vi "总磷总氮断电保存全局变量.vi"() -> ()   [LabVIEW 2022 SP3, in "斯坦道氨氮V2.lvlib"]
panel:
  in  "命令格式":u16(ring)=2 items=["自动", "低位在前", "低位在后"]
  in  "波特率":u32(ring)=115200 items=["115200"=115200, "9600"=9600]
  in  "低量程上限":cluster{"总磷":dbl, "总氮":dbl, "氨氮":dbl}={"总磷"=1.0, "总氮"=10.0, "氨氮"=1.0}
  out "总氮消解温度":dbl=120.0 caption="消解时长："
  out "总磷消解温度":dbl=120.0 caption="消解时长："
  out "校准条件":cluster{"线性相关系数":dbl}={"线性相关系数"=0.999}
  out "总氮消解时长":dbl=30.0 caption="消解时长："
  out "总磷消解时长":dbl=30.0 caption="消解时长："
  in  "盐度自动补偿：":bool
  out "启动队列名称":cluster{"String":string, "Value":u16}[](array[cluster])
  in  "氨氮自动测试量程配置":T1={"水样测试量程模式"=enum."AUTO", "空白核查量程模式"=enum."AUTO", "跨度核查量程模式"=enum."AUTO", "加标回收量程模式"=enum."AUTO", "标样核查量程模式"=enum."AUTO"}
  in  "MB通信方式选择":enum16{"串口", "TCP"}(ring)
  in  "PORT":string="502"
  in  "IP":string
  in  "VISA Resource":refnum<visa-resource-name>
  in  "运行周期":T2={"运行模式"=enum."维护模式", "质控频次"=enum."关闭", "空白核查时间"=2, "跨度核查时间"=6, "测量间隔"=240.0} {"跨度核查时间" items=["00H", "01H", "02H", "03H", "04H", "05H", "06H", "07H", "08H", "09H", "10H", "11H", "12H", "13H", "14H", "15H", "16H", "17H", "18H", "19H", "20H", "21H", "22H", "23H", "关闭"]; "空白核查时间" items=["00H", "01H", "02H", "03H", "04H", "05H", "06H", "07H", "08H", "09H", "10H", "11H", "12H", "13H", "14H", "15H", "16H", "17H", "18H", "19H", "20H", "21H", "22H", "23H", "关闭"]}
  in  "流程路径":path=path "data/流程.xml"
  in  "总氮自动测试量程配置":T1={"水样测试量程模式"=enum."AUTO", "空白核查量程模式"=enum."AUTO", "跨度核查量程模式"=enum."AUTO", "加标回收量程模式"=enum."AUTO", "标样核查量程模式"=enum."AUTO"}
  in  "质控参数设置":T3
  in  "总磷自动测试量程配置":T1={"水样测试量程模式"=enum."AUTO", "空白核查量程模式"=enum."AUTO", "跨度核查量程模式"=enum."AUTO", "加标回收量程模式"=enum."AUTO", "标样核查量程模式"=enum."AUTO"}
  # "℃"
  # "℃"
  # "min"
  # "min"
  # "运行模式："
  # "质控频次："
  # "零点核查时间："
  # "跨度核查时间："
  # "质控参数设置"
  # "总氮"
  # "氨氮"
  # "监测参数"
  # "总磷"
  # "跨度值"
  # "零点核查标准液浓度"
  # "跨度核查标准液浓度"
  # "标样核查标准液浓度"
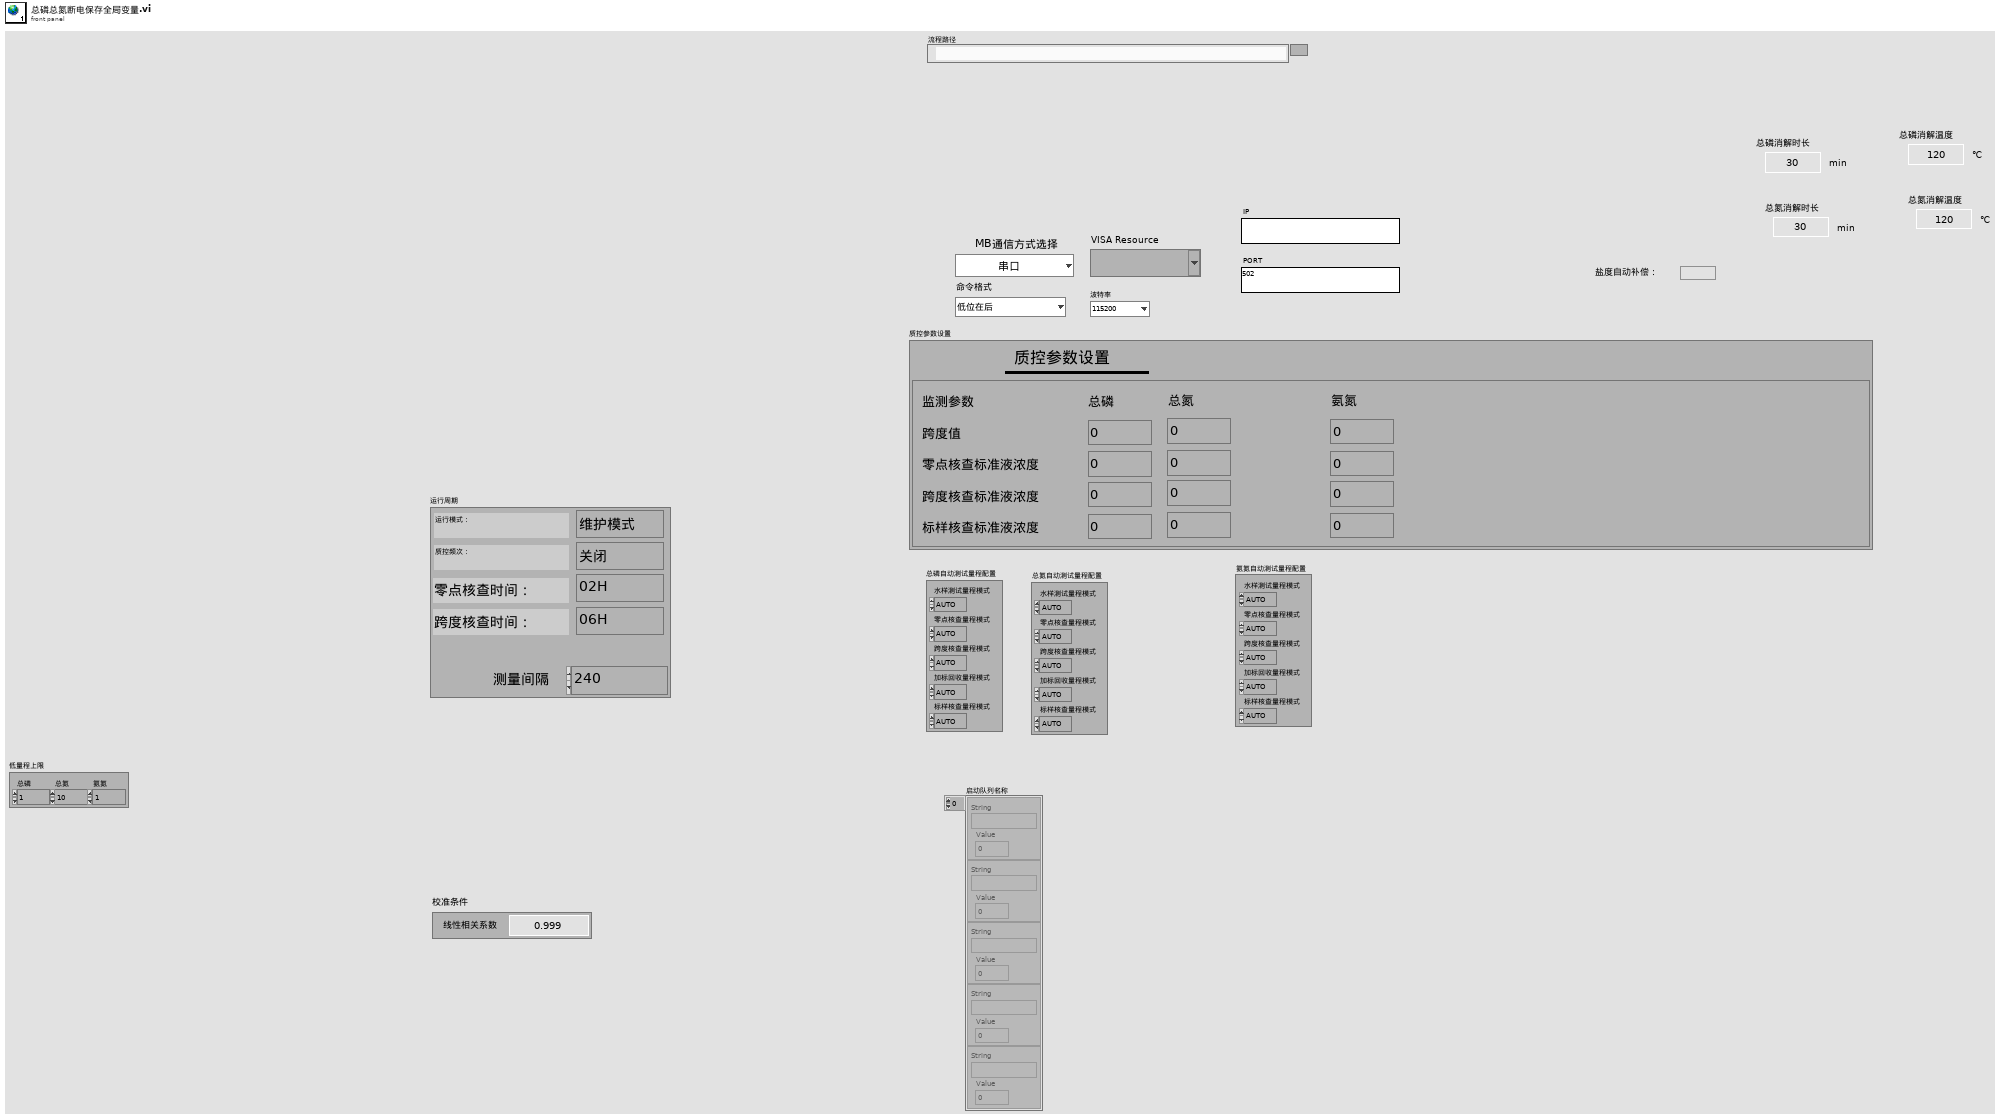
[diagram p1: front panel]
types:
  T1 = cluster{"水样测试量程模式":enum16{"H", "L", "AUTO"}, "空白核查量程模式":enum16{"H", "L", "AUTO"}, "跨度核查量程模式":enum16{"H", "L", "AUTO"}, "加标回收量程模式":enum16{"H", "L", "AUTO"}, "标样核查量程模式":enum16{"H", "L", "AUTO"}}
  T2 = cluster{"运行模式":enum16{"维护模式", "常规模式", "应急模式", "质控模式", "性能测试"}, "质控频次":enum16{"关闭", "每天", "星期一", "星期二", "星期三", "星期四", "星期五", "星期六", "星期日"}, "空白核查时间":u16, "跨度核查时间":u16, "测量间隔":dbl}
  T3 = cluster{"总磷跨度值":dbl, "总磷零点标准液浓度":dbl, "总磷跨度标准液浓度":dbl, "总磷标准液标准浓度":dbl, "总氮跨度值":dbl, "总氮零点标准液浓度":dbl, "总氮跨度标准液浓度":dbl, "总氮标准液标准浓度":dbl, "氨氮跨度值":dbl, "氨氮零点标准液浓度":dbl, "氨氮跨度标准液浓度":dbl, "氨氮标准液标准浓度":dbl}
diagram:
